vi "Config info.vi"() -> (1 "info com":cluster{"PORT":string, "BAUDRATE":string}, 2 "info database":T1)   [LabVIEW 2015]
uses:
  <vilib>/Utility/config.llb/Write Key (String).vi
  <vilib>/Utility/config.llb/Read Key (String).vi
  <vilib>/Utility/config.llb/NI_LVConfig.lvlib
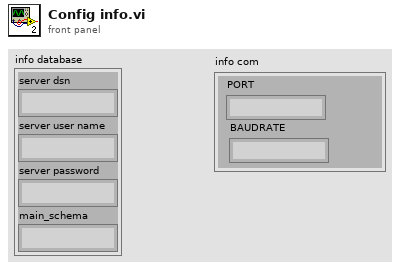
[diagram p1: front panel]
types:
  T1 = cluster{"server dsn":string, "server user name":string, "server password":string, "main_schema":string}
  T2 = typedef "NI_LVConfig.lvlib/Config Data RefNum.ctl" = refnum<k1>
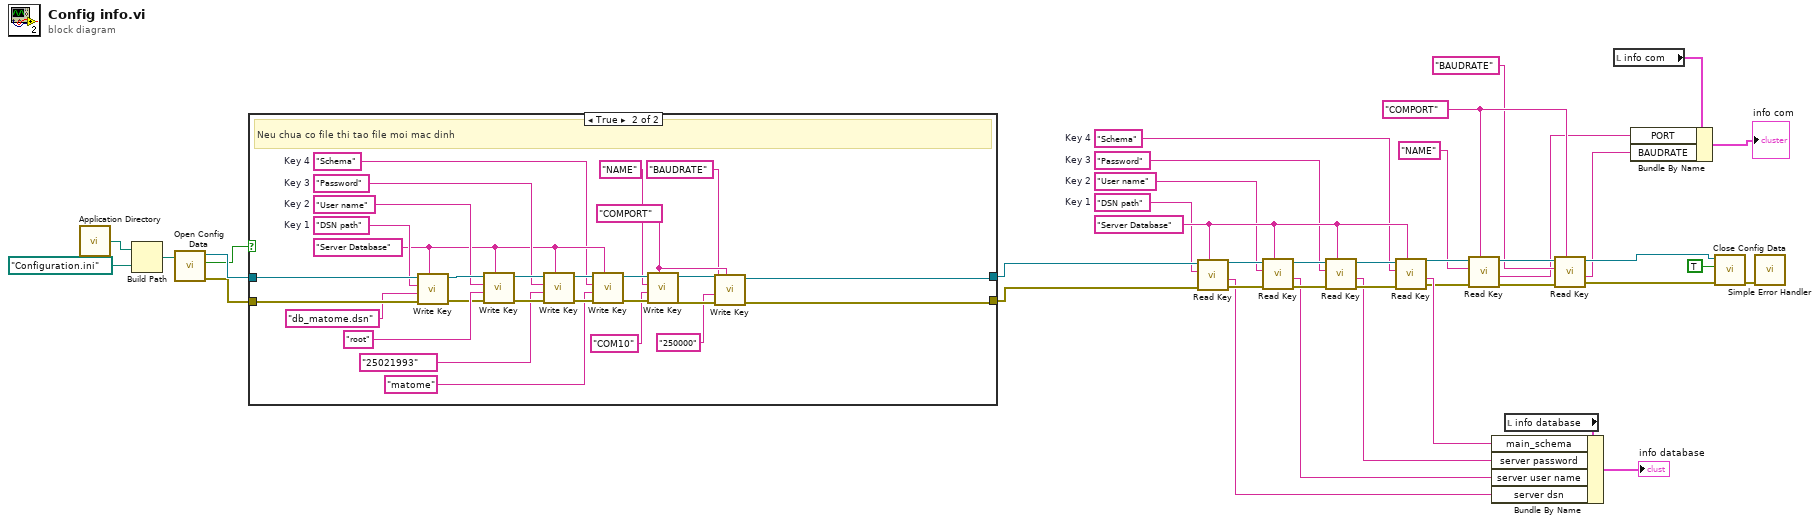
[diagram p0: block diagram]
diagram:
  w7 = "COMPORT" ("section")
  w20 = "Schema"  # Key 4
  w21 = "Password"  # Key 3
  w22 = "User name"  # Key 2
  w23 = "DSN path"  # Key 1
  w24 = "Server Database"
  n1 = call <vilib>:"Application Directory.vi"() -> ("Application Directory"=w27:path)
  n2 = Build Path(base path=w27, name or relative path=path "Configuration.ini" ("default name")) -> (appended path=w39:path)
  n3 = call <vilib>:"Open Config Data.vi"("configuration file path"=w39) -> ("error out"=w37:errorcluster, "file created?"=w34:bool, "refnum"=w38:T2)  [unwired: 2 in, 6 out]
  n4 = case shown="True" w34 {
    tunnel: w38 -> [w42 w65]
    tunnel: w37 -> [w41 w66]
    tunnel: [w42 w44] -> w33
    tunnel: [w41 w43] -> w32
    frame False {
    }
    frame True {
      w51 = "COMPORT" ("section")
      w56 = "Schema"  # Key 4
      w62 = "Password"  # Key 3
      w61 = "User name"  # Key 2
      w60 = "DSN path"  # Key 1
      w57 = "Server Database"
      # "Neu chua co file thi tao file moi mac dinh"
      n5 = call-poly <vilib>:"Write Key.vi"("section"=w57, "error in (no error)"=w66, "value"="db_matome.dsn", "key"=w60, "refnum"=w65) -> ("error out"=w63:errorcluster, "refnum out"=w64:T2)  [unwired: 4 in, 1 out]
      n6 = call-poly <vilib>:"Write Key.vi"("section"=w57, "error in (no error)"=w63, "value"="root", "key"=w61, "refnum"=w64) -> ("error out"=w70:errorcluster, "refnum out"=w69:T2)  [unwired: 1 in, 4 out]
      n7 = call-poly <vilib>:"Write Key.vi"("section"=w57, "error in (no error)"=w70, "value"="25021993", "key"=w62, "refnum"=w69) -> ("error out"=w59:errorcluster, "refnum out"=w58:T2)  [unwired: 1 in, 4 out]
      n8 = call-poly <vilib>:"Write Key.vi"("section"=w57, "error in (no error)"=w59, "value"="matome", "key"=w56, "refnum"=w58) -> ("error out"=w53:errorcluster, "refnum out"=w52:T2)  [unwired: 1 in, 4 out]
      n9 = call-poly <vilib>:"Write Key.vi"("section"=w51, "error in (no error)"=w53, "value"="COM10", "key"="NAME", "refnum"=w52) -> ("error out"=w47:errorcluster, "refnum out"=w48:T2)  [unwired: 1 in, 4 out]
      n10 = call-poly <vilib>:"Write Key.vi"("section"=w51, "error in (no error)"=w47, "value"="250000", "key"="BAUDRATE", "refnum"=w48) -> ("error out"=w43:errorcluster, "refnum out"=w44:T2)  [unwired: 1 in, 4 out]
    }
  }
  n11 = call-poly <vilib>:"Read Key.vi"("section"=w24, "error in (no error)"=w32, "key"=w23, "refnum"=w33) -> ("error out"=w30:errorcluster, "value"=w17:string, "refnum out"=w31:T2)  [unwired: 4 in, 1 out]
  n12 = call-poly <vilib>:"Read Key.vi"("section"=w24, "error in (no error)"=w30, "key"=w22, "refnum"=w31) -> ("error out"=w29:errorcluster, "value"=w16:string, "refnum out"=w28:T2)  [unwired: 2 in, 3 out]
  n13 = call-poly <vilib>:"Read Key.vi"("section"=w24, "error in (no error)"=w29, "key"=w21, "refnum"=w28) -> ("error out"=w25:errorcluster, "value"=w15:string, "refnum out"=w26:T2)  [unwired: 2 in, 3 out]
  n14 = call-poly <vilib>:"Read Key.vi"("section"=w24, "error in (no error)"=w25, "key"=w20, "refnum"=w26) -> ("error out"=w8:errorcluster, "value"=w14:string, "refnum out"=w12:T2)  [unwired: 2 in, 3 out]
  n15 = call-poly <vilib>:"Read Key.vi"("section"=w7, "error in (no error)"=w8, "key"="NAME", "refnum"=w12) -> ("error out"=w9:errorcluster, "value"=w2:string, "refnum out"=w13:T2)  [unwired: 2 in, 3 out]
  n16 = local read "info database"() -> (w19:T1)
  n17 = Bundle By Name(cluster=w19, "main_schema"=w14, "server password"=w15, "server user name"=w16, "server dsn"=w17) -> (→"info database":T1)
  n18 = call-poly <vilib>:"Read Key.vi"("section"=w7, "error in (no error)"=w9, "key"="BAUDRATE", "refnum"=w13) -> ("error out"=w10:errorcluster, "value"=w1:string, "refnum out"=w11:T2)  [unwired: 2 in, 3 out]
  n19 = local read "info com"() -> (w3:cluster{"PORT":string, "BAUDRATE":string})
  n20 = Bundle By Name(cluster=w3, "PORT"=w2, "BAUDRATE"=w1) -> (→"info com":cluster{"PORT":string, "BAUDRATE":string})
  n21 = call <vilib>:"Close Config Data.vi"("error in (no error)"=w10, "write file if changed (T)"=TRUE ("write configuration file? (T)"), "refnum"=w11) -> ("error out"=w36:errorcluster)  [unwired: 8 out]
  n22 = call <vilib>:"Simple Error Handler.vi"("error in (no error)"=w36) -> ()  [unwired: 1 in, 8 out]
